vi "read_location.vi"(8 "error in (no error)":errorcluster, 11 "TempProbe in":refnum<class "TempProbe.lvclass">) -> (0 "error out":errorcluster, 2 "Location":string, 3 "TempProbe out":refnum<class "TempProbe.lvclass">)   [LabVIEW 2010, in "TempProbe.lvclass"]
uses:
  TempProbe.lvclass
  TempProbe.lvclass/TempProbe.ctl
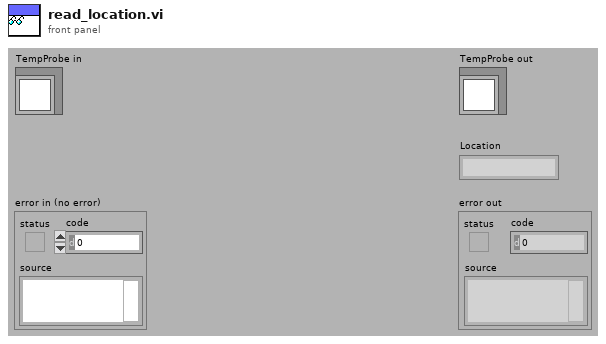
[diagram p1: front panel]
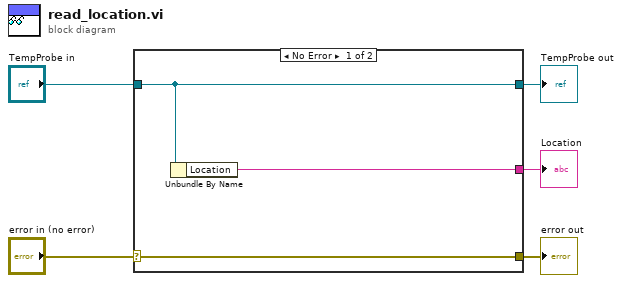
[diagram p0: block diagram]
diagram:
  n1 = case shown="No Error" "error in (no error)" {
    selector: "error in (no error)" -> [w8 w9]
    tunnel: [w8 w9] -> w4
    tunnel: [w7 w10] -> w2
    tunnel: "TempProbe in" -> [w7 w10]
    tunnel: [w6 _] -> w1
    frame No Error {
      n2 = Unbundle By Name(w7) -> ("Location"=w6:string)
    }
    frame Error {
    }
  }
  "error out" <- w4
  "TempProbe out" <- w2
  "Location" <- w1
